vi "StressTest.vi"() -> ()   [LabVIEW 2009]
panel:
  out "Data out":string
  out "error out":errorcluster
  out "Iterations":i32
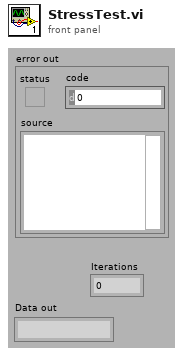
[diagram p1: front panel]
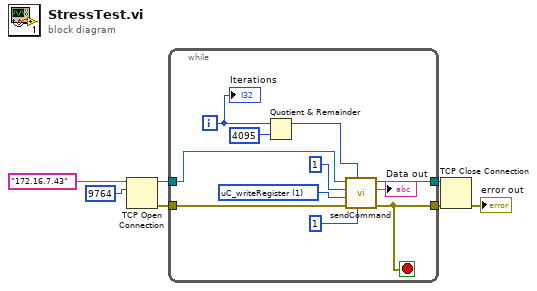
[diagram p0: block diagram]
diagram:
  n1 = TCP Open Connection(address="172.16.7.43", remote port or service name=u16 9764) -> (connection ID=w7:refnum<k5>, error out=w4:errorcluster)  [unwired: 3 in]
  n2 = while {
    tunnel: w7 -> [w15]
    tunnel: w4 -> [w16]
    tunnel: [w9] -> w3
    tunnel: [w14] -> w2
    i -> [w11]
    stop <- w9 stop-if-true
    w17 = u16 1 items=["sendCommand"=9, "FPGA_writeRegister"=3, "FPGA_readRegister"=2, "uC_writeRegister"=1, "uC_readRegister"=0] ("Action")
    n3 = Quotient & Remainder(x=w11, y=4095) -> (x-y*floor(x/y)=w10:i32)  [unwired: 1 out]
    n4 = call "sendCommand.vi"("Address"=1, "Data"=w10, "error in"=w16, "Action"=w17, "id_in"=1 ("id"), "connection ID"=w15) -> ("error out"=w9:errorcluster, "Data out"=→"Data out":string, "connection ID out"=w14:refnum<k5>)  [unwired: 1 in, 2 out]
    "Iterations" <- w11
  }
  n5 = TCP Close Connection(connection ID=w2, error in (no error)=w3) -> (error out=→"error out":errorcluster)  [unwired: 1 in, 1 out]
